vi "Profile Loop.vi"(11 "FPGA Ref":T1) -> ()   [LabVIEW 2019]
uses:
  Controls/FPGA_Reference.ctl
  <vilib>/Platform/TimedLoop/XDataNode/timing_clust.ctl
  <vilib>/Platform/TimedLoop/XDataNode/nitl_modes.ctl
  <vilib>/Platform/TimedLoop/XDataNode/wakeup.ctl
  <vilib>/Utility/error.llb/Error Cluster From Error Code.vi
  <vilib>/rvi/errors/niLvFpgaAdjustHostInterfaceError.vi
  <vilib>/Platform/TimedLoop/XDataNode/XDataNode.xnode
  <vilib>/rvi/interface/nirviReadWriteControl/nirviReadWriteControl.xnode
  FPGA Bitfiles/TI sbRIO Main (FPGA, 9627).lvbitx
  FPGA/TI sbRIO Main (FPGA).vi
  <vilib>/Platform/TimedLoop/XDataNode/XDNodeRunTimeDep.lvlib
  NiFpgaLv.dll
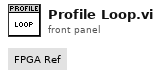
[diagram p1: front panel]
types:
  T1 = typedef "FPGA_Reference.ctl" = refnum<k20>
  T2 = typedef "XDNodeRunTimeDep.lvlib/timing_clust.ctl" = cluster{"Expected End [f-1]":u64, "Actual End [f-1]":u64, "Finished Late? [f-1]":bool, "Expected End [i-1]":u64, "Actual End [i-1]":u64, "Finished Late? [i-1]":bool, "Expected Start [i]":u64, "Actual Start [i]":u64, "Expected Start [f]":u64, "Actual Start [f]":u64, "Source Name":string, "Structure Name":string, "Period":i64, "Deadline":i64, "Offset":i64, "Start":i64, "Priority":i32, "Timeout":i32, "Mode":T3, "Wakeup Reason":T4, "Error":errorcluster, "Source Type":string, "Secondary Source Type":string, "Global End Time":u64, "Global Start Time":u64, "Frame Duration":u64, "Iteration Duration":u64, "Assigned CPU":i32, "I/O Scan Engine Mode":u32}
  T3 = typedef "XDNodeRunTimeDep.lvlib/nitl_modes.ctl" = enum32{"No Change", "Process missed periods, maintain original phase", "Discard missed periods, maintain original phase", "Process missed periods, ignore original phase", "Discard missed periods, ignore original phase"}
  T4 = typedef "XDNodeRunTimeDep.lvlib/wakeup.ctl" = enum32{"Normal", "Aborted", "Asynchronous wakeup", "Timing source error", "Timed loop error", "Timeout"}
  T5 = typedef "Test Step (FPGA).ctl" = cluster{"Step":u8, "Time (ms)":u32, "Target\nSpeed":u16, "Pump Cmds (Ticks)":i32[], "Pump Cmds (Duty)":u32[], "Relays":bool[], "PS Cmd":fxp<+/-,20,5>, "Pressure Cmd":fxp<+/-,20,5>, "Temp\nCmd":i16}
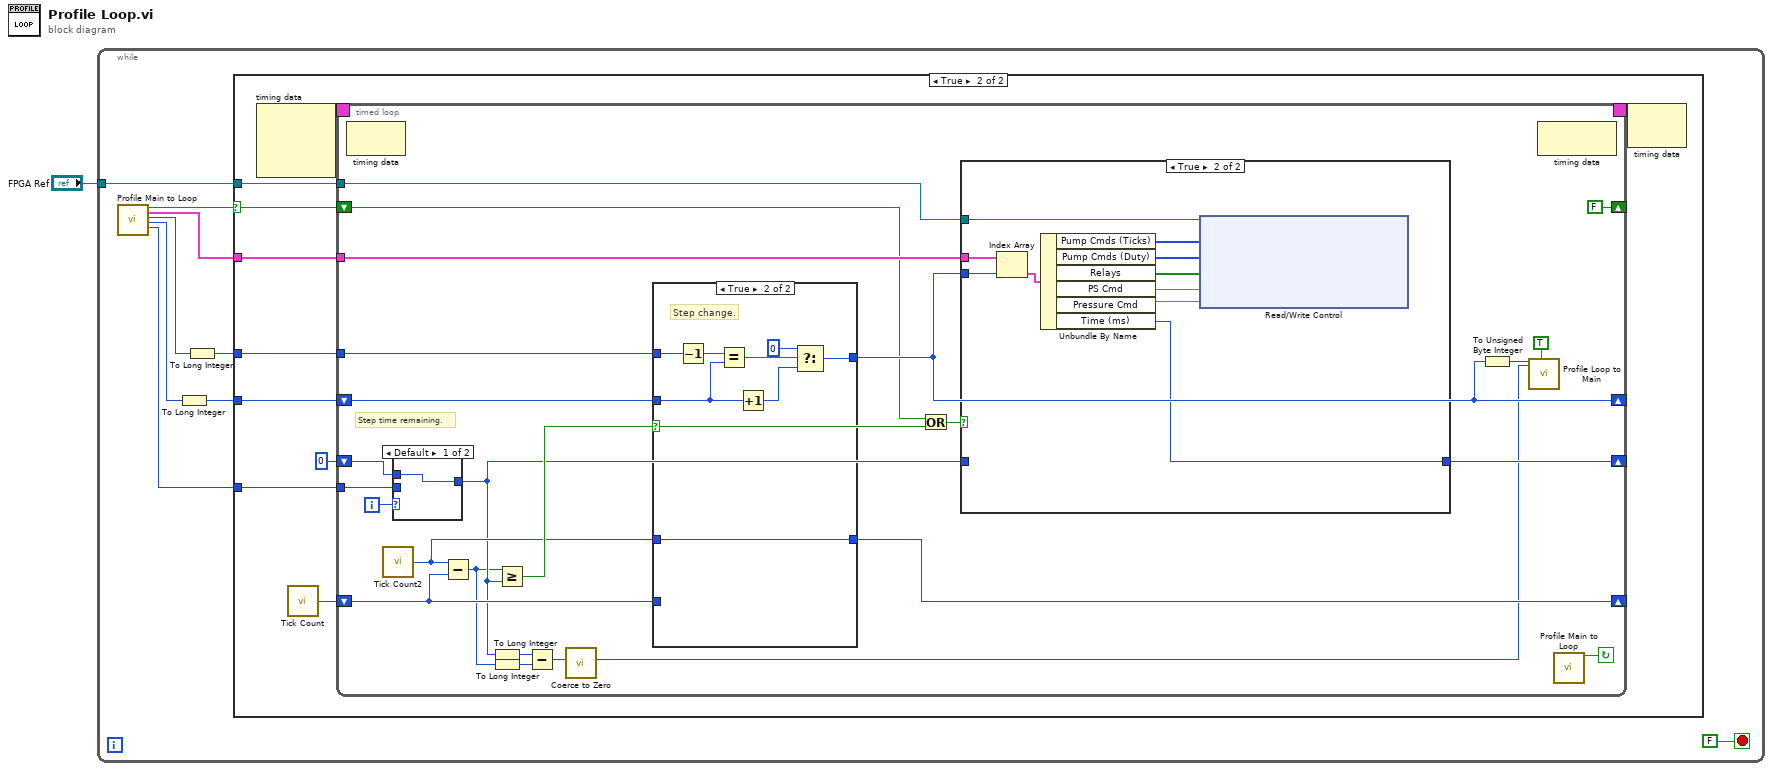
[diagram p0: block diagram]
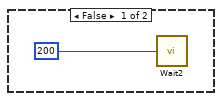
[diagram p2: hidden frame]
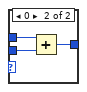
[diagram p3: hidden frame]
diagram:
  n1 = while {
    tunnel: "FPGA Ref" -> [w3]
    stop <- FALSE stop-if-true
    n2 = call "Profile Main to Loop.vi"() -> ("Run Profile OUT"=w7:bool, "Test Profile (FPGA) OUT"=w6:T5[], "Profile Steps OUT"=w5:u8, "Current Step OUT"=w4:u8, "Step Time Left OUT"=w2:u32)  [unwired: 14 in, 1 out]
    n3 = To Long Integer(number=w4) -> (32bit integer=w9:i32)
    n4 = To Long Integer(number=w5) -> (32bit integer=w8:i32)
    n5 = case shown="True" w7 {
      selector: w7 -> [_ w17]
      tunnel: w6 -> [_ w21]
      tunnel: w9 -> [_ w20]
      tunnel: w8 -> [_ w19]
      tunnel: w3 -> [_ w18]
      tunnel: w2 -> [_ w15]
      frame False {
        n6 = call "Wait2"("Count(mSec)"=u32 200) -> ()  [unwired: 1 out]
      }
      frame True {
        n7 = node-c288() -> (w13:T2)  [unwired: 3 in]
        n8 = call "Tick Count"() -> ("Tick Count(mSec)"=w14:u32)
        n9 = timed-loop {
          tunnel: w21 -> [w46]
          shift-right: [w44] -> _
          shift-left: w20 -> [w45]
          shift-right: [w35] -> _
          shift-left: u32 0 ("Time (ms)") -> [w32]
          tunnel: w19 -> [w43]
          tunnel: w18 -> [w41]
          shift-right: [FALSE] -> _
          shift-left: w17 -> [w39]
          tunnel: w15 -> [w33]
          shift-right: [w29] -> _
          shift-left: w14 -> [w28]
          timing: w13 -> [_]
          timing-out: [_] -> w12
          i -> [w34]
          stop <- w42 continue-if-true
          # "Step time remaining."
          n10 = node-c288() -> ()  [unwired: 1 in, 1 out]
          n11 = call "Tick Count2"() -> ("Tick Count(mSec)"=w30:u32)
          n12 = case shown="Default" w34 {
            tunnel: w32 -> [w49 w52]
            tunnel: w33 -> [_ w51]
            tunnel: [w49 w50] -> w27
            frame Default {
            }
            frame 0 {
              n13 = Add(x=w52, y=w51) -> (x+y=w50:u32)
            }
          }
          n14 = Subtract(x=w30, y=w28) -> (x-y=w26:u32)
          n15 = To Long Integer(number=w27) -> (32bit integer=w25:i32)
          n16 = To Long Integer(number=w26) -> (32bit integer=w24:i32)
          n17 = Greater Or Equal?(x=w26, y=w27) -> (x >= y?=w31:bool)
          n18 = Subtract(x=w25, y=w24) -> (x-y=w23:i32)
          n19 = call "Coerce to Zero.vi"("Number IN"=w23) -> ("Number OUT"=w22:i32)  [unwired: 10 in]
          n20 = case shown="True" w31 {
            tunnel: w43 -> [_ w73]
            tunnel: w45 -> [w65 w70]
            tunnel: [w65 w67] -> w44
            tunnel: [w64 w66] -> w29
            tunnel: w30 -> [_ w66]
            tunnel: w28 -> [w64 _]
            frame False {
            }
            frame True {
              # "Step change."
              n21 = Decrement(x=w73) -> (x-1=w72:i32)
              n22 = Equal?(x=w72, y=w70) -> (x = y?=w71:bool)
              n23 = Increment(x=w70) -> (x+1=w69:i32)
              n24 = Select(t=0, s=w71, f=w69) -> (s? t:f=w67:i32)
            }
          }
          n25 = Or(x=w39, y=w31) -> (x .or. y?=w38:bool)
          n26 = case shown="True" w38 {
            tunnel: w46 -> [_ w63]
            tunnel: w44 -> [_ w61]
            tunnel: [w53 w56] -> w35
            tunnel: w41 -> [_ w60]
            tunnel: w27 -> [w53 _]
            frame False {
            }
            frame True {
              n27 = Index Array(array=w63, index=w61) -> (element=w62:T5)
              n28 = Unbundle By Name(w62) -> ("Pump Cmds (Ticks)"=w55:i32[], "Pump Cmds (Duty)"=w54:u32[], "Relays"=w59:bool[], "PS Cmd"=w58:fxp<+/-,20,5>, "Pressure Cmd"=w57:fxp<+/-,20,5>, "Time (ms)"=w56:u32)
              n29 = xnode "Read/Write Control"("FPGA VI Reference In"=w60, "Duty (Ticks)"=w55, "Pump Cmds (Duty)"=w54, "Power Relays"=w59, "PS Cmd"=w58, "Pressure Cmd"=w57) -> ()  [unwired: 1 in, 2 out]
            }
          }
          n30 = To Unsigned Byte Integer(number=w44) -> (unsigned 8bit integer=w37:u8)
          n31 = call "Profile Loop to Main.vi"("Current Step"=w37, "Step Time Left"=w22, "Write (F)"=TRUE) -> ()  [unwired: 15 in, 2 out]
          n32 = node-c288() -> ()  [unwired: 1 in, 1 out]
          n33 = call "Profile Main to Loop.vi"() -> ("Run Profile OUT"=w42:bool)  [unwired: 14 in, 5 out]
        }
        n34 = node-c288(w12) -> ()  [unwired: 1 out]
      }
    }
  }
